vi "ziGetValueAuxIn.vi"(3 "error in":errorcluster, 4 "Path":string, 5 "Handle In":T2 {"Handle" format="0x%08x"; "Conn" format="0x%08x"}) -> (0 "error out":errorcluster, 1 "AuxIn Value":T1, 2 "Handle Out":T2 {"Handle" format="0x%08x"; "Conn" format="0x%08x"})   [LabVIEW 2018, in "Zurich Instruments LabOne.lvlib"]
doc: "This vi retrieves the newest available AUXin sample from the specified node. The vi returns the value first found if more than one value is available (a wildcard is used in the Path)."
uses:
  Zurich Instruments LabOne.lvlib
  <instrlib>/Zurich Instruments LabOne/Private/ziLV64.framework
  ziTypeHandle.ctl
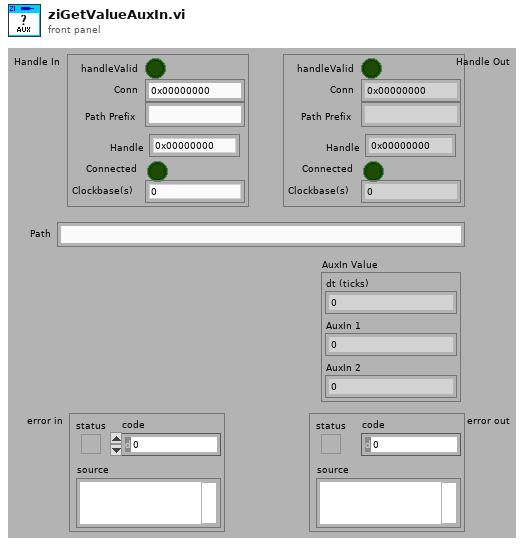
[diagram p1: front panel]
types:
  T1 = cluster{"dt (ticks)":u64, "AuxIn 1":dbl, "AuxIn 2":dbl}
  T2 = typedef "Zurich Instruments LabOne.lvlib/ziTypeHandle.ctl" = cluster{"handleValid":bool, "Conn":u64, "Path Prefix":string, "Handle":u64, "Connected":bool, "Clockbase(s)":dbl}
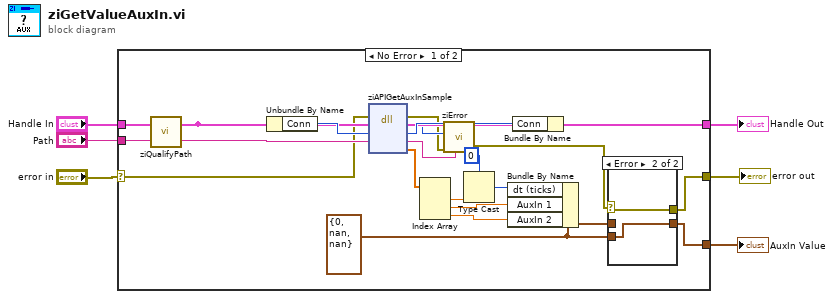
[diagram p0: block diagram]
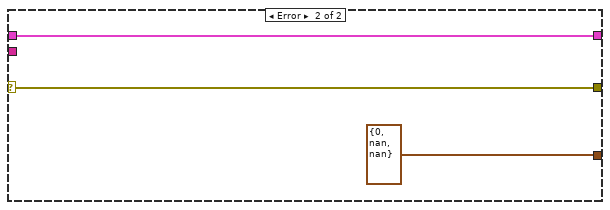
[diagram p3: hidden frame]
diagram:
  n1 = case shown="No Error" "error in" {
    selector: "error in" -> [w18 w35]
    tunnel: [w28 w34] -> w6
    tunnel: [w15 T1 {"dt (ticks)"=0, "AuxIn 1"=nan, "AuxIn 2"=nan} ("AuxIn Value 2")] -> w5
    tunnel: "Path" -> [w22 _]
    tunnel: "Handle In" -> [w21 w34]
    tunnel: [w13 w35] -> w2
    frame No Error {
      w12 = T1 {"dt (ticks)"=0, "AuxIn 1"=nan, "AuxIn 2"=nan} ("AuxIn Value 2")
      n2 = call "ziQualifyPath.vi"("Path In"=w22, "Handle In"=w21) -> ("Path Out"=w23:string, "Handle Out"=w24:T2)
      n3 = Unbundle By Name(w24) -> ("Conn"=w27:u64)
      n4 = dll-call lib="Applications/National Instruments/LabVIEW 2019 64-bit/instr.lib/Zurich Instruments LabOne/Private/ziLV*.*" fn="ziAPIGetAuxInSample"(error in=w18, "Conn"=w27, "Path"=w23) -> (error out=w19:errorcluster, "return type"=w20:u32, "Conn"=w26:u64, "Path"=w17:string, "AuxinSample"=w25:dbl[])  [unwired: 2 in, 2 out]
      n5 = Index Array(array=w25) -> (element #1=w9:dbl, element #2=w11:dbl, element #3=w10:dbl)  [unwired: 3 in]
      n6 = call "ziError.vi"("ziErrorCode"=w20, "Error In"=w19, "Annotation"=w17) -> ("Error Out"=w14:errorcluster)  [unwired: 3 in]
      n7 = Type Cast(type=u64 0 ("DIO"), x=w9) -> (*(type *) &x=w8:u64)
      n8 = Bundle By Name(cluster=w12, "dt (ticks)"=w8, "AuxIn 1"=w11, "AuxIn 2"=w10) -> (w16:T1)
      n9 = Bundle By Name(cluster=w24, "Conn"=w26) -> (w28:T2)
      n10 = case shown="Error" w14 {
        selector: w14 -> [w29 w31]
        tunnel: w16 -> [w30 _]
        tunnel: [w30 w32] -> w15
        tunnel: w12 -> [_ w32]
        tunnel: [w29 w31] -> w13
        frame No Error {
        }
        frame Error {
        }
      }
    }
    frame Error {
    }
  }
  "Handle Out" <- w6
  "error out" <- w2
  "AuxIn Value" <- w5
